vi "WSVCAP SHL Host LL I2C Convert 4 Bytes to Status and Capacitance.vi"(0 "C:1-64 Read Data [U8]":u8[][](array[numeric]) format="%.0x") -> (4 "AD7747 Values":string[][](table))   [LabVIEW 2017]
panel:
  out "Data Headers":u8[](array[numeric])=[1, 2, 3, 4, 5, 6, 7, 8, 9, 10, 11, 12, 12, 14, 15, 16, 17, 18, 19, 20, 21, 22, 23, 24, 25, 26, 27, 28, 29, 30, 31, 32, 33, 34, 35, 36]
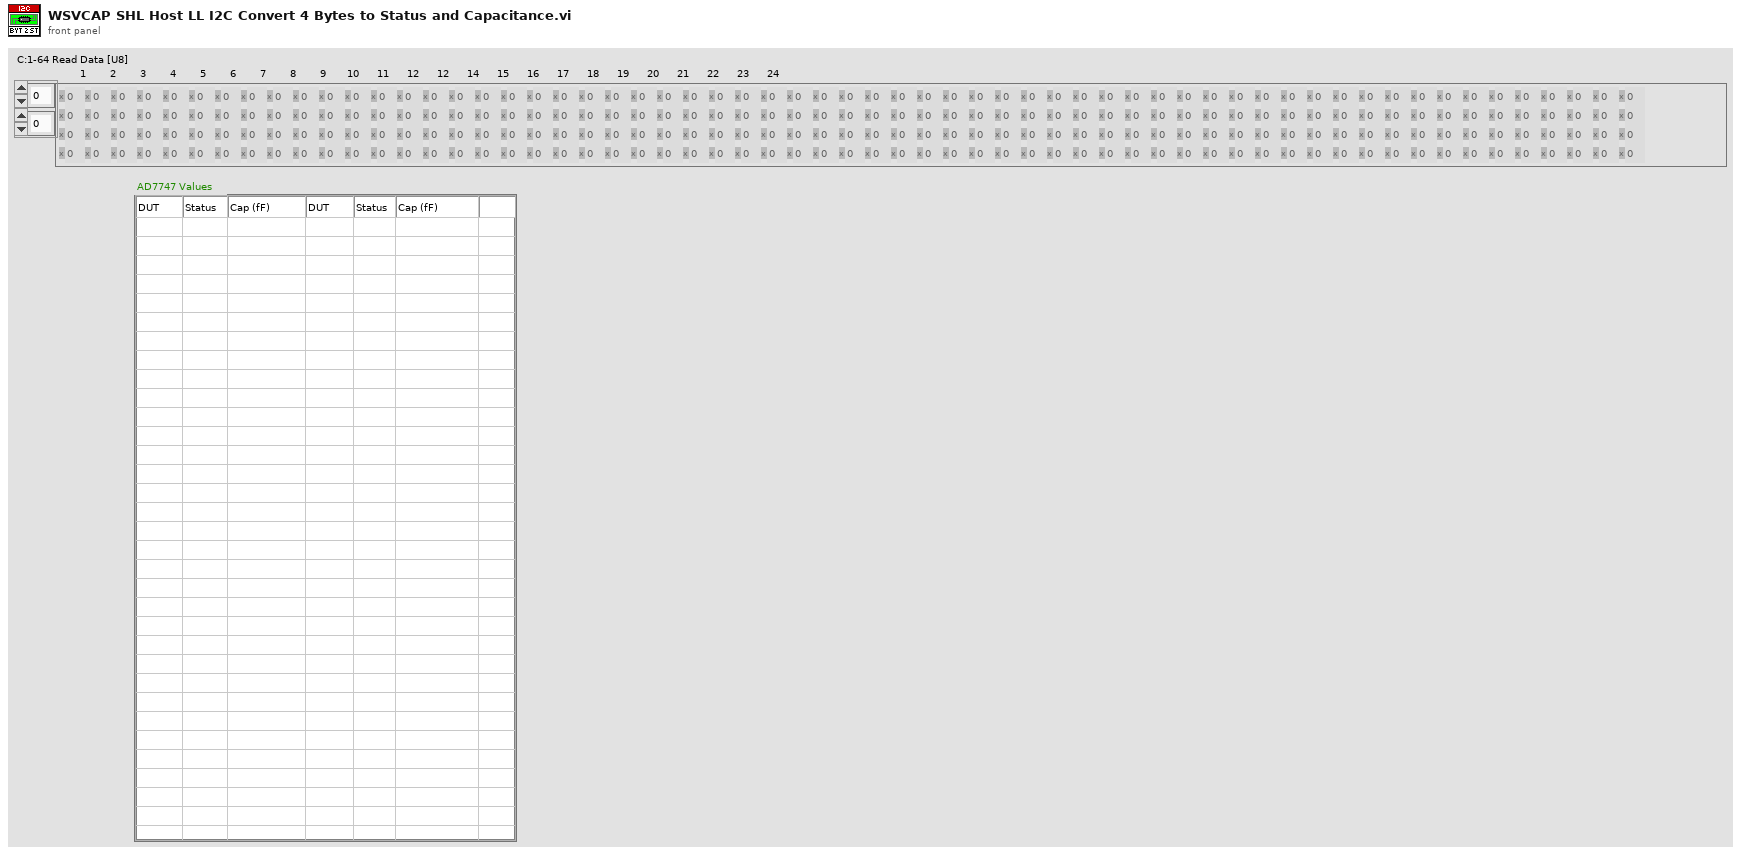
[diagram p1: front panel]
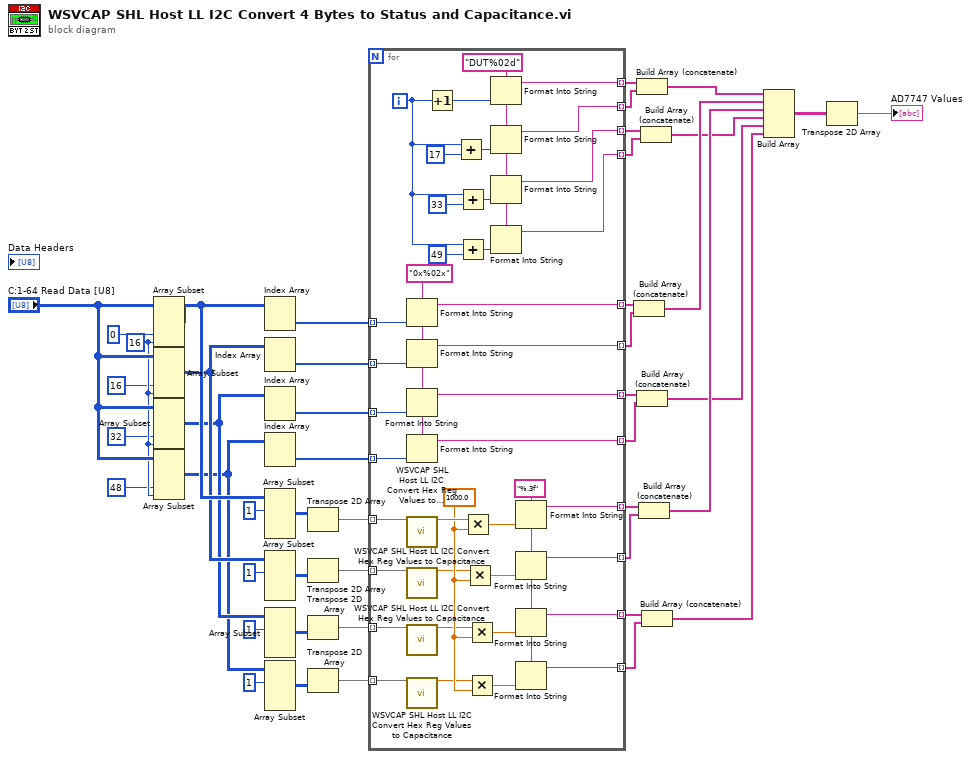
[diagram p0: block diagram]
diagram:
  w28 = 16 ("length")
  n1 = Array Subset(array="C:1-64 Read Data [U8]", index (col)=0 ("length"), length (col)=w28) -> (w29:u8[][])  [unwired: 2 in]
  n2 = Array Subset(array="C:1-64 Read Data [U8]", index (col)=16 ("length"), length (col)=w28) -> (w23:u8[][])  [unwired: 2 in]
  n3 = Array Subset(array="C:1-64 Read Data [U8]", index (col)=32 ("length"), length (col)=w28) -> (w22:u8[][])  [unwired: 2 in]
  n4 = Array Subset(array="C:1-64 Read Data [U8]", index (col)=48 ("length"), length (col)=w28) -> (w21:u8[][])  [unwired: 2 in]
  n5 = Index Array(array=w29) -> (element=w45:u8[])  [unwired: 2 in]
  n6 = Index Array(array=w23) -> (element=w46:u8[])  [unwired: 2 in]
  n7 = Index Array(array=w22) -> (element=w35:u8[])  [unwired: 2 in]
  n8 = Index Array(array=w21) -> (element=w31:u8[])  [unwired: 2 in]
  n9 = Array Subset(array=w29, index (row)=1 ("index")) -> (w42:u8[][])  [unwired: 3 in]
  n10 = Array Subset(array=w23, index (row)=1 ("index")) -> (w41:u8[][])  [unwired: 3 in]
  n11 = Array Subset(array=w22, index (row)=1 ("index")) -> (w37:u8[][])  [unwired: 3 in]
  n12 = Array Subset(array=w21, index (row)=1 ("index")) -> (w33:u8[][])  [unwired: 3 in]
  n13 = Transpose 2D Array(2D array=w42) -> (transposed array=w40:u8[][])
  n14 = Transpose 2D Array(2D array=w41) -> (transposed array=w39:u8[][])
  n15 = Transpose 2D Array(2D array=w37) -> (transposed array=w38:u8[][])
  n16 = Transpose 2D Array(2D array=w33) -> (transposed array=w32:u8[][])
  n17 = for {
    tunnel: w46 -> [w83] mode=indexing
    tunnel: w45 -> [w84] mode=indexing
    tunnel: w40 -> [w86] mode=indexing
    tunnel: w39 -> [w85] mode=indexing
    tunnel: [w82] -> w16 mode=indexing
    tunnel: [w81] -> w12 mode=indexing
    tunnel: [w80] -> w15 mode=indexing
    tunnel: [w79] -> w11 mode=indexing
    tunnel: w38 -> [w77] mode=indexing
    tunnel: [w78] -> w10 mode=indexing
    tunnel: w35 -> [w76] mode=indexing
    tunnel: [w75] -> w14 mode=indexing
    tunnel: w32 -> [w74] mode=indexing
    tunnel: [w73] -> w9 mode=indexing
    tunnel: w31 -> [w71] mode=indexing
    tunnel: [w72] -> w13 mode=indexing
    tunnel: [w60] -> w20 mode=indexing
    tunnel: [w59] -> w19 mode=indexing
    tunnel: [w58] -> w18 mode=indexing
    tunnel: [w57] -> w17 mode=indexing
    i -> [w67]
    w54 = 1000.0 ("y")
    w56 = "DUT%02d" ("format string")
    w69 = "%.3f" ("format string")
    w70 = "0x%02x" ("format string")
    n18 = Format Into String(format string=w70, w84) -> (resulting string=w82:string)  [unwired: 2 in, 1 out]
    n19 = Format Into String(format string=w70, w83) -> (resulting string=w80:string)  [unwired: 2 in, 1 out]
    n20 = Format Into String(format string=w70, w76) -> (resulting string=w75:string)  [unwired: 2 in, 1 out]
    n21 = Format Into String(format string=w70, w71) -> (resulting string=w72:string)  [unwired: 2 in, 1 out]
    n22 = call "WSVCAP SHL Host LL I2C Convert Hex Reg Values to Capacitance.vi"("Bytes (H-M-L)"=w86) -> ("Capacitance (pF)"=w55:dbl)  [unwired: 14 in]
    n23 = call "WSVCAP SHL Host LL I2C Convert Hex Reg Values to Capacitance.vi"("Bytes (H-M-L)"=w85) -> ("Capacitance (pF)"=w51:dbl)  [unwired: 14 in]
    n24 = call "WSVCAP SHL Host LL I2C Convert Hex Reg Values to Capacitance.vi"("Bytes (H-M-L)"=w77) -> ("Capacitance (pF)"=w52:dbl)  [unwired: 14 in]
    n25 = call "WSVCAP SHL Host LL I2C Convert Hex Reg Values to Capacitance.vi"("Bytes (H-M-L)"=w74) -> ("Capacitance (pF)"=w53:dbl)  [unwired: 14 in]
    n26 = Increment(x=w67) -> (x+1=w68:i32)
    n27 = Add(x=w67, y=17) -> (x+y=w63:i32)
    n28 = Add(x=w67, y=33) -> (x+y=w62:i32)
    n29 = Add(x=w67, y=49) -> (x+y=w61:i32)
    n30 = Multiply(x=w55, y=w54) -> (x*y=w50:dbl)
    n31 = Multiply(x=w51, y=w54) -> (x*y=w49:dbl)
    n32 = Multiply(x=w52, y=w54) -> (x*y=w48:dbl)
    n33 = Multiply(x=w53, y=w54) -> (x*y=w47:dbl)
    n34 = Format Into String(format string=w56, w68) -> (resulting string=w60:string)  [unwired: 2 in, 1 out]
    n35 = Format Into String(format string=w56, w63) -> (resulting string=w59:string)  [unwired: 2 in, 1 out]
    n36 = Format Into String(format string=w56, w62) -> (resulting string=w58:string)  [unwired: 2 in, 1 out]
    n37 = Format Into String(format string=w56, w61) -> (resulting string=w57:string)  [unwired: 2 in, 1 out]
    n38 = Format Into String(format string=w69, w50) -> (resulting string=w81:string)  [unwired: 2 in, 1 out]
    n39 = Format Into String(format string=w69, w49) -> (resulting string=w79:string)  [unwired: 2 in, 1 out]
    n40 = Format Into String(format string=w69, w48) -> (resulting string=w78:string)  [unwired: 2 in, 1 out]
    n41 = Format Into String(format string=w69, w47) -> (resulting string=w73:string)  [unwired: 2 in, 1 out]
  }
  n42 = Build Array (concatenate)(w16, w15) -> (w7:string[])
  n43 = Build Array (concatenate)(w20, w19) -> (w8:string[])
  n44 = Build Array (concatenate)(w14, w13) -> (w4:string[])
  n45 = Build Array (concatenate)(w12, w11) -> (w6:string[])
  n46 = Build Array (concatenate)(w18, w17) -> (w5:string[])
  n47 = Build Array (concatenate)(w10, w9) -> (w3:string[])
  n48 = Build Array(w8, w7, w6, w5, w4, w3) -> (w2:string[][])
  n49 = Transpose 2D Array(2D array=w2) -> (transposed array=→"AD7747 Values":string[][])
